vi "State Enter.vi"(11 "Destroying Self Actor State in":refnum<class "Destroying Self Actor State.lvclass">) -> (0 "error out":errorcluster, 3 "Destroying Self Actor State out":refnum<class "Destroying Self Actor State.lvclass">)   [LabVIEW 2021, in "LVCAM.lvlib" / "Destroying Self Actor State.lvclass"]
uses:
  Destroying Self Actor State.lvclass
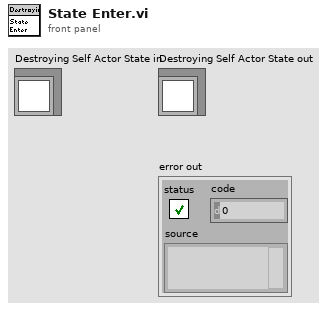
[diagram p1: front panel]
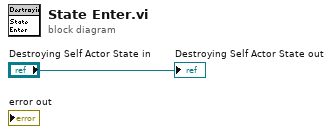
[diagram p0: block diagram]
diagram:
  "Destroying Self Actor State out" <- "Destroying Self Actor State in"
